vi "Update.vi"(8 "error in (no error)":errorcluster, 11 "Duck in":refnum<class "Duck.lvclass">) -> (0 "error out":errorcluster, 2 "Variant":variant, 3 "Duck out":refnum<class "Duck.lvclass">)   [LabVIEW 2013, in "Duck.lvclass"]
uses:
  Duck.lvclass
  Observer.lvclass/Observer.lvclass
  Duck.lvclass/Duck.ctl
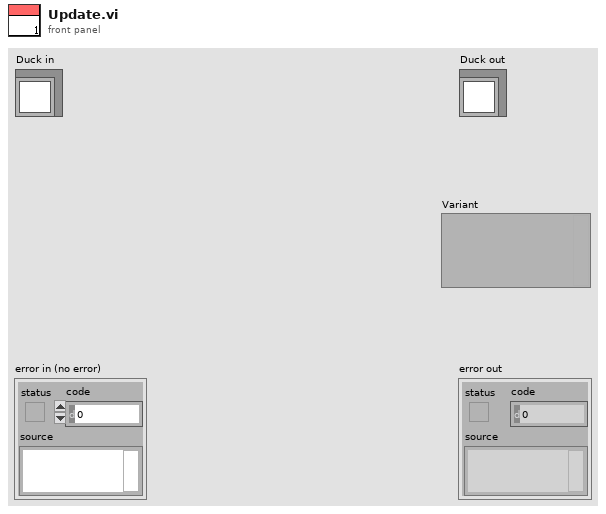
[diagram p1: front panel]
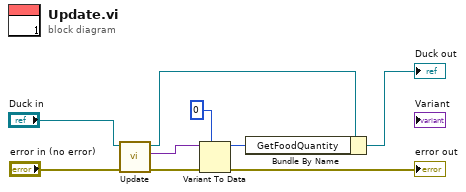
[diagram p0: block diagram]
diagram:
  n1 = call-parent "Update.vi"("error in (no error)"="error in (no error)", "Observer in"="Duck in") -> ("error out"=w4:errorcluster, "Variant"=w6:variant, "Observer out"=w7:refnum<class "Duck.lvclass">)  [unwired: 7 in]
  n2 = Variant To Data(error in=w4, type=0, Variant=w6) -> (data=w2:i32, error out=→"error out":errorcluster)
  n3 = Bundle By Name(cluster=w7, "GetFoodQuantity"=w2) -> (→"Duck out":refnum<class "Duck.lvclass">)
